vi "8 Ch Digital Output.vi"(2 "Packet":u64, 4 "8 Ch Digital Out":T1={"DO0"="Chassis2/Mod2/DO0", "DO1"="Chassis2/Mod2/DO1", "DO2"="Chassis2/Mod2/DO2", "DO3"="Chassis2/Mod2/DO3", "DO4"="Chassis2/Mod1/DO4", "DO5"="Chassis2/Mod2/DO5", "DO6"="Chassis2/Mod2/DO6", "DO7"="Chassis2/Mod2/DO7"}) -> ()   [LabVIEW 2009]
uses:
  <vilib>/eio/EIONode/EIONode.xnode
  <vilib>/rvi/eio/nirviEIOImplementation/nirviEIOImplementation.xnode
  <vilib>/rvi/eio/common/nirviEmuTemplateMethod_noerrors.vi
  <vilib>/rvi/eio/common/nirviEmuClasses.ctl
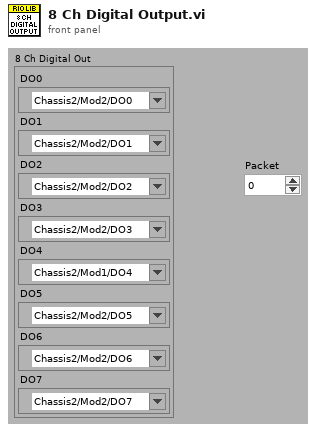
[diagram p1: front panel]
types:
  T1 = cluster{"DO0":refnum<k21>, "DO1":refnum<k21>, "DO2":refnum<k21>, "DO3":refnum<k21>, "DO4":refnum<k21>, "DO5":refnum<k21>, "DO6":refnum<k21>, "DO7":refnum<k21>}
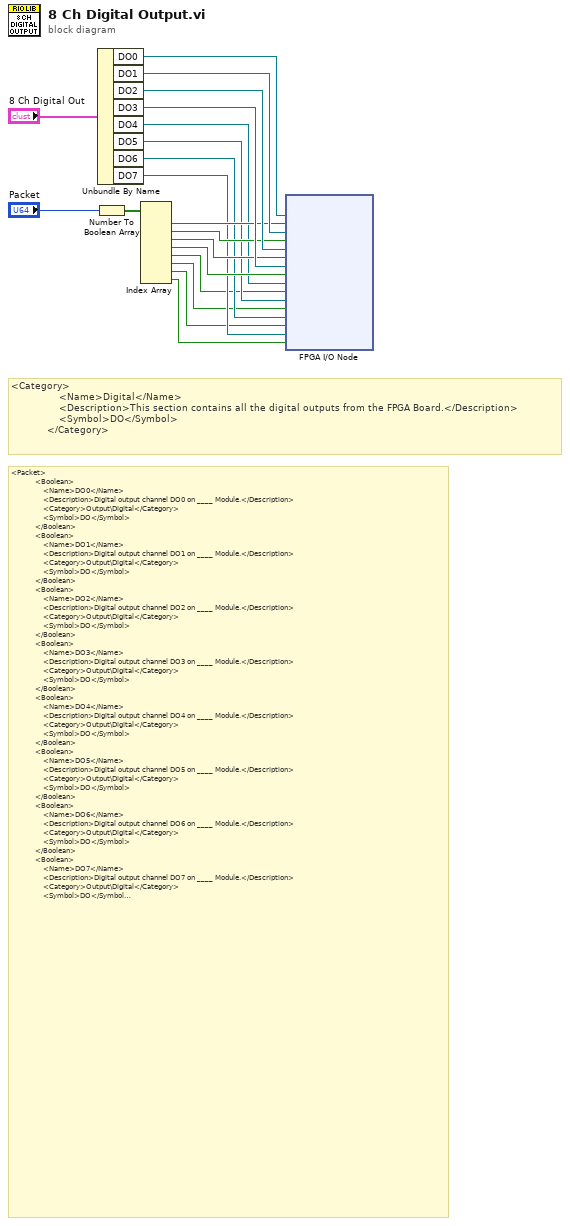
[diagram p0: block diagram]
diagram:
  # "<Category>\n                <Name>Digital</Name>\n                <Description>This section contains all the digital outputs from the FPGA Board.</Description>\n                <Symbol>DO</Symbol>\n            </Category>"
  # "<Packet>\n            <Boolean>\n                <Name>DO0</Name>\n                <Description>Digital output channel DO0 on ____ Module.</Description>\n                <Category>Output\\Digital</Category>\n                <Symbol>DO</Symbol>\n            </Boolean>\n            <Boolean>\n                <Name>DO1</Name>\n                <Description>Digital output channel DO1 on ____ Module.</Description>\n                <Category>Output\\Digital</Category>\n                <Symbol>DO</Symbol>\n            </Boolean>\n            <Boolean>\n                <Name>DO2</Name>\n                <Description>Digital output channel DO2 on ____ Module.</Description>\n                <Category>Output\\Digital</Category>\n                <Symbol>DO</Symbol>\n            </Boolean>\n            <Boolean>\n                <Name>DO3</Name>\n                <Description>Digital output channel DO3 on ____ Module.</Description>\n                <Category>Output\\Digital</Category>\n                <Symbol>DO</Symbol>\n            </Boolean>\n            <Boolean>\n                <Name>DO4</Name>\n                <Description>Digital output channel DO4 on ____ Module.</Description>\n                <Category>Output\\Digital</Category>\n                <Symbol>DO</Symbol>\n            </Boolean>\n            <Boolean>\n                <Name>DO5</Name>\n                <Description>Digital output channel DO5 on ____ Module.</Description>\n                <Category>Output\\Digital</Category>\n                <Symbol>DO</Symbol>\n            </Boolean>\n            <Boolean>\n                <Name>DO6</Name>\n                <Description>Digital output channel DO6 on ____ Module.</Description>\n                <Category>Output\\Digital</Category>\n                <Symbol>DO</Symbol>\n            </Boolean>\n            <Boolean>\n                <Name>DO7</Name>\n                <Description>Digital output channel DO7 on ____ Module.</Description>\n                <Category>Output\\Digital</Category>\n                <Symbol>DO</Symbol>\n            </Boolean>\n        </Packet>"
  n1 = Number To Boolean Array(number="Packet") -> (Boolean array=w10:bool[])
  n2 = Unbundle By Name("8 Ch Digital Out") -> ("DO0"=w16:refnum<k21>, "DO1"=w19:refnum<k21>, "DO2"=w18:refnum<k21>, "DO3"=w17:refnum<k21>, "DO4"=w8:refnum<k21>, "DO5"=w7:refnum<k21>, "DO6"=w6:refnum<k21>, "DO7"=w5:refnum<k21>)
  n3 = Index Array(array=w10) -> (element #1=w11:bool, element #2=w14:bool, element #3=w13:bool, element #4=w12:bool, element #5=w1:bool, element #6=w2:bool, element #7=w3:bool, element #8=w4:bool)  [unwired: 8 in]
  n4 = xnode "FPGA I/O Node"("I/O Item"=w11, "I/O Item"=w14, "I/O Item"=w13, "I/O Item"=w12, "I/O Item"=w1, "I/O Item"=w2, "I/O Item"=w3, "I/O Item"=w4, "FPGA I/O In"=w16, "FPGA I/O In"=w19, "FPGA I/O In"=w18, "FPGA I/O In"=w17, "FPGA I/O In"=w8, "FPGA I/O In"=w7, "FPGA I/O In"=w6, "FPGA I/O In"=w5) -> ()  [unwired: 8 out]
